vi "MALT Open.vi"(8 "error in":errorcluster, 10 "port":u16=2013, 11 "address":string) -> (0 "error out":errorcluster={"status"=TRUE, "code"=0, "source"="Nem sikerült megnyitni a TCP kapcsolatot"})   [LabVIEW 2018]
uses:
  Private/Global/MALT Global.vi
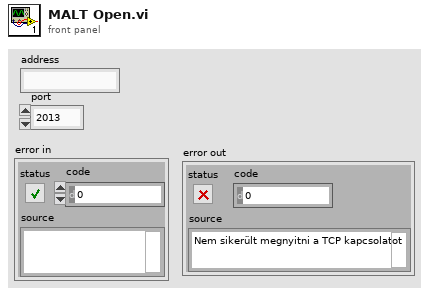
[diagram p1: front panel]
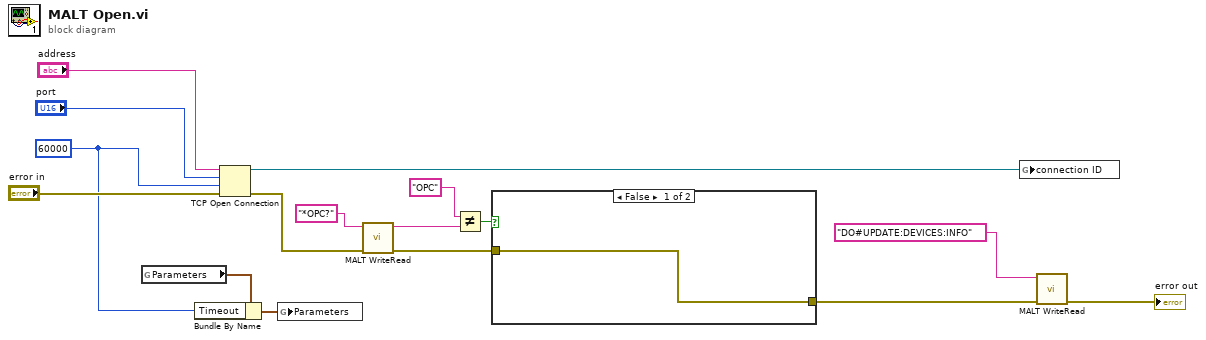
[diagram p0: block diagram]
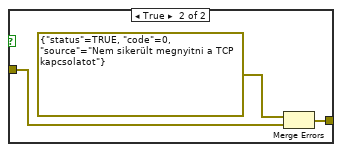
[diagram p2: hidden frame]
diagram:
  w11 = 60000 ("timeout ms (60000)")
  n1 = global read "MALT Global.vi" "Parameters"() -> (w12:cluster{"Timeout":i32})
  n2 = Bundle By Name(cluster=w12, "Timeout"=w11) -> (w10:cluster{"Timeout":i32})
  n3 = TCP Open Connection(address="address", remote port or service name="port", timeout ms (60000)=w11, error in (no error)="error in") -> (connection ID=w13:refnum<k5>, error out=w9:errorcluster)  [unwired: 1 in]
  n4 = global write "MALT Global.vi" "Parameters"(w10) -> ()
  n5 = call "MALT WriteRead.vi"("error in"=w9, "Request"="*OPC?" ("data in")) -> ("error out"=w6:errorcluster, "Response"=w4:string)  [unwired: 8 in]
  n6 = Not Equal?(x="OPC", y=w4) -> (x != y?=w7:bool)
  n7 = case shown="False" w7 {
    tunnel: w6 -> [w17 w20]
    tunnel: [w17 w18] -> w3
    frame False {
    }
    frame True {
      n8 = Merge Errors(errorcluster {"status"=TRUE, "code"=0, "source"="Nem sikerült megnyitni a TCP kapcsolatot"} ("error in"), w20) -> (w18:errorcluster)
    }
  }
  n9 = global write "MALT Global.vi" "connection ID"(w13) -> ()
  n10 = call "MALT WriteRead.vi"("error in"=w3, "Request"="DO#UPDATE:DEVICES:INFO" ("data in")) -> ("error out"=→"error out":errorcluster)  [unwired: 8 in, 1 out]
